vi "data_processor.vi"(0 "Active Analog Data Packages In":T1[](array[typedef]), 1 "start time":timestamp=timestamp(3643888167.3510303 s since 1904-01-01), 5 "data":waveform(dbl)[](array[waveform]), 11 "error in":errorcluster) -> (4 "Analog Data Array":T1[](array[typedef]), 10 "timestamp":dbl[](array[numeric])=[11.30071570032691, 11.30121570032691, 11.301715700326909, 11.30221570032691, 11.30271570032691, 11.30321570032691, 11.30371570032691, 11.30421570032691, 11.30471570032691, 11.30521570032691, 11.30571570032691, 11.30621570032691, 11.30671570032691, 11.30721570032691, 11.30771570032691, 11.30821570032691, 11.308715700326909, 11.30921570032691, 11.30971570032691, 11.310215700326909, 11.31071570032691, 11.31121570032691, 11.311715700326909, 11.31221570032691, 11.31271570032691, 11.313215700326909, 11.31371570032691, 11.31421570032691, 11.314715700326909, 11.31521570032691, 11.31571570032691, 11.316215700326909, 11.31671570032691, 11.31721570032691, 11.317715700326909, 11.31821570032691, 11.31871570032691, 11.31921570032691, 11.31971570032691, 11.32021570032691, 11.32071570032691, 11.32121570032691, 11.321715700326909, 11.32221570032691, 11.32271570032691, 11.323215700326909, 11.32371570032691, 11.32421570032691, 11.324715700326909, 11.32521570032691, 11.32571570032691, 11.326215700326909, 11.32671570032691, 11.32721570032691, 11.327715700326909, 11.32821570032691, 11.32871570032691, 11.329215700326909, 11.32971570032691, 11.33021570032691, 11.330715700326909, 11.33121570032691, 11.33171570032691, 11.332215700326909, 11.33271570032691, 11.33321570032691, 11.33371570032691, 11.33421570032691, 11.33471570032691, 11.33521570032691, 11.33571570032691, 11.33621570032691, 11.33671570032691, 11.33721570032691, 11.33771570032691, 11.33821570032691, 11.33871570032691, 11.339215700326909, 11.33971570032691, 11.34021570032691, 11.340715700326909, 11.34121570032691, 11.34171570032691, 11.342215700326909, 11.34271570032691, 11.34321570032691, 11.343715700326909, 11.34421570032691, 11.34471570032691, 11.345215700326909, 11.34571570032691, 11.34621570032691, 11.346715700326909, 11.34721570032691, 11.34771570032691, 11.348215700326909, 11.34871570032691, 11.34921570032691, 11.34971570032691, 11.35021570032691, 11.35071570032691, 11.35121570032691, 11.35171570032691, 11.35221570032691, 11.35271570032691, 11.35321570032691, 11.353715700326909, 11.35421570032691, 11.35471570032691, 11.355215700326909, 11.35571570032691, 11.35621570032691, 11.356715700326909, 11.35721570032691, 11.35771570032691, 11.358215700326909, 11.35871570032691, 11.35921570032691, 11.359715700326909, 11.36021570032691, 11.36071570032691, 11.361215700326909, 11.36171570032691, 11.36221570032691, 11.362715700326909, 11.36321570032691, 11.36371570032691, 11.364215700326909, 11.36471570032691, 11.36521570032691, 11.36571570032691, 11.36621570032691, 11.36671570032691, 11.36721570032691, 11.36771570032691, 11.36821570032691, 11.36871570032691, 11.36921570032691, 11.36971570032691, 11.37021570032691, 11.37071570032691, 11.371215700326909, 11.37171570032691, 11.37221570032691, 11.372715700326909, 11.37321570032691, 11.37371570032691, 11.374215700326909, 11.37471570032691, 11.37521570032691, 11.375715700326909, 11.37621570032691, 11.37671570032691, 11.377215700326909, 11.37771570032691, 11.37821570032691, 11.378715700326909, 11.37921570032691, 11.37971570032691, 11.380215700326909, 11.38071570032691, 11.38121570032691, 11.38171570032691, 11.38221570032691, 11.38271570032691, 11.38321570032691, 11.38371570032691, 11.384215700326909, 11.38471570032691, 11.38521570032691, 11.385715700326909, 11.38621570032691, 11.38671570032691, 11.387215700326909, 11.38771570032691, 11.38821570032691, 11.388715700326909, 11.38921570032691, 11.38971570032691, 11.390215700326909, 11.39071570032691, 11.39121570032691, 11.391715700326909, 11.39221570032691, 11.39271570032691, 11.393215700326909, 11.39371570032691, 11.39421570032691, 11.394715700326909, 11.39521570032691, 11.39571570032691, 11.39621570032691, 11.39671570032691, 11.39721570032691, 11.39771570032691, 11.39821570032691, 11.39871570032691, 11.39921570032691, 11.39971570032691, 11.40021570032691], 14 "Number of Points":i32=200, 15 "error out":errorcluster)   [LabVIEW 2017]
uses:
  <vilib>/gmath/NI_Gmath.lvlib
  <vilib>/Analysis/NI_AALBase.lvlib
  <vilib>/Analysis/baseanly.llb/Mean (DBL).vi
  <vilib>/Waveform/WDTOps.llb/WDT Get Waveform Time Array DBL.vi
  analog_data.ctl
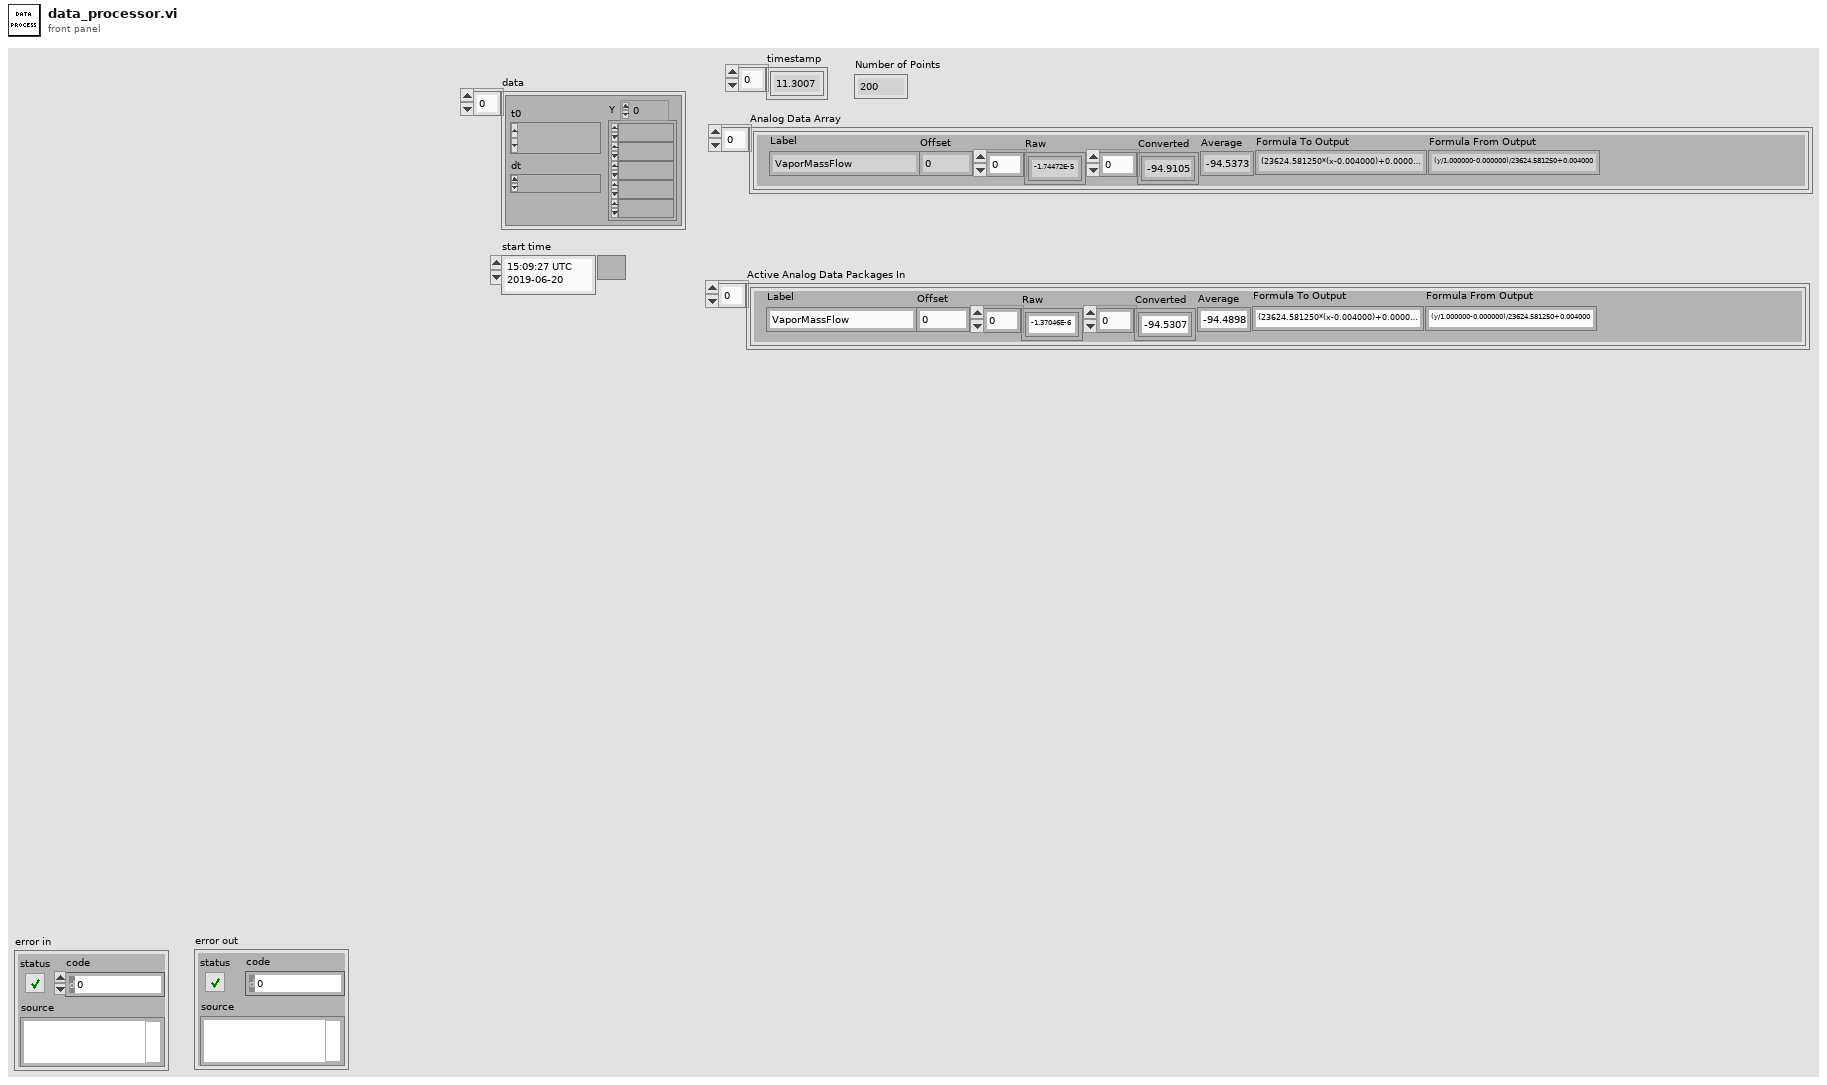
[diagram p1: front panel]
types:
  T1 = typedef "analog_data.ctl" = cluster{"Label":string, "Offset":dbl, "Raw":dbl[], "Converted":dbl[], "Average":dbl, "Formula To Output":string, "Formula From Output":string}
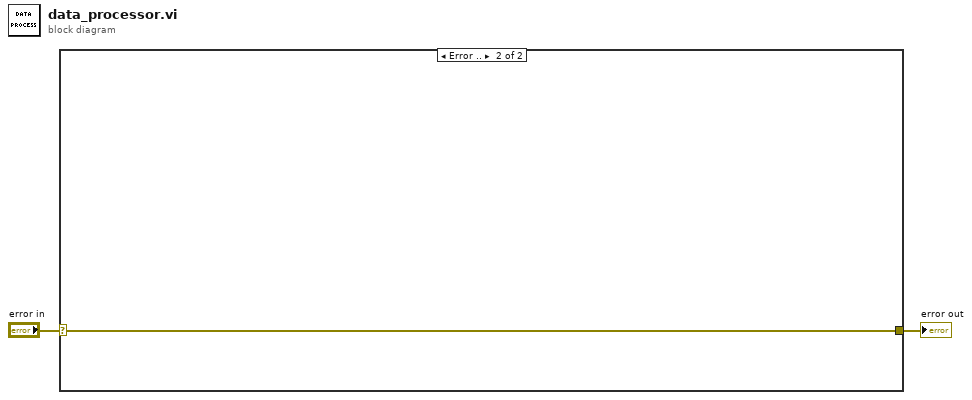
[diagram p0: block diagram]
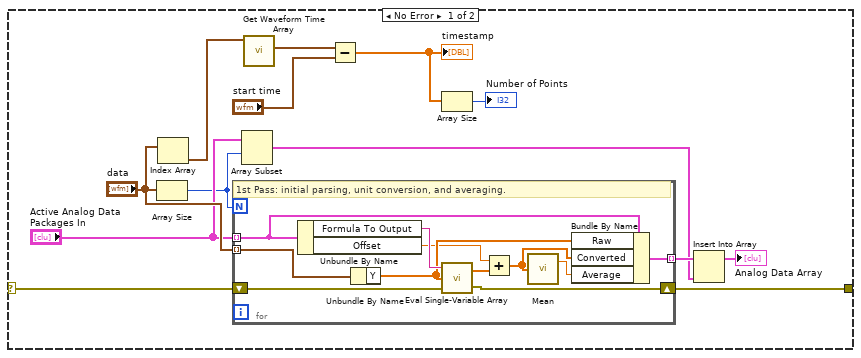
[diagram p2: hidden frame]
diagram:
  n1 = case shown="Error .." "error in" {
    selector: "error in" -> [w3 w27]
    tunnel: [w15 w27] -> w2
    frame No Error {
      n2 = Array Size(array="data") -> (size(s)=w7:i32)
      n3 = Index Array(array="data") -> (element=w11:waveform(dbl))  [unwired: 1 in]
      n4 = for {
        N: w7 -> [_]
        tunnel: "Active Analog Data Packages In" -> [w16] mode=indexing
        tunnel: "data" -> [w26] mode=indexing
        tunnel: [w19] -> w10 mode=indexing
        shift-right: [w18] -> w15
        shift-left: w3 -> [w17]
        # "1st Pass: initial parsing, unit conversion, and averaging."
        n5 = Unbundle By Name(w16) -> ("Formula To Output"=w25:string, "Offset"=w20:dbl)
        n6 = Unbundle By Name(w26) -> ("Y"=w24:dbl[])
        n7 = call <vilib>:"Eval Single-Variable Array.vi"("error in (no error)"=w17, "X Values"=w24, "formula"=w25) -> ("error out"=w18:errorcluster, "Y Values"=w22:dbl[])
        n8 = Add(x=w20, y=w22) -> (x+y=w21:dbl[])
        n9 = call-poly <vilib>:"Mean.vi"("X"=w21) -> ("mean"=w23:dbl)  [unwired: 1 out]
        n10 = Bundle By Name(cluster=w16, "Raw"=w24, "Converted"=w21, "Average"=w23) -> (w19:T1)
      }
      n11 = Array Subset(array="Active Analog Data Packages In", index=w7) -> (w6:T1[])  [unwired: 1 in]
      n12 = call-poly <vilib>:"Get Waveform Time Array.vi"("waveform in"=w11) -> ("X array"=w14:timestamp[])  [unwired: 9 in, 1 out]
      n13 = Subtract(x=w14, y="start time") -> (x-y=w5:dbl[])
      "timestamp" <- w5
      n14 = Array Size(array=w5) -> (size(s)=→"Number of Points":i32)
      n15 = Insert Into Array(array=w10, new element=w6) -> (→"Analog Data Array":T1[])  [unwired: 1 in]
    }
    frame Error {
    }
  }
  "error out" <- w2
